vi "Serial_Read_String.vi"(8 "error in (no error)":errorcluster, 11 "VISA Refnum in":refnum<visa-resource-name>) -> (0 "error out":errorcluster, 2 "read buffer":string, 3 "VISA Refnum out":refnum<visa-resource-name>)   [LabVIEW 2020]
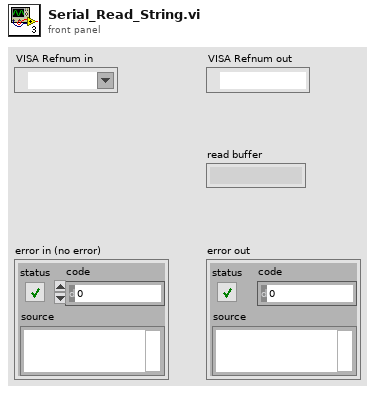
[diagram p1: front panel]
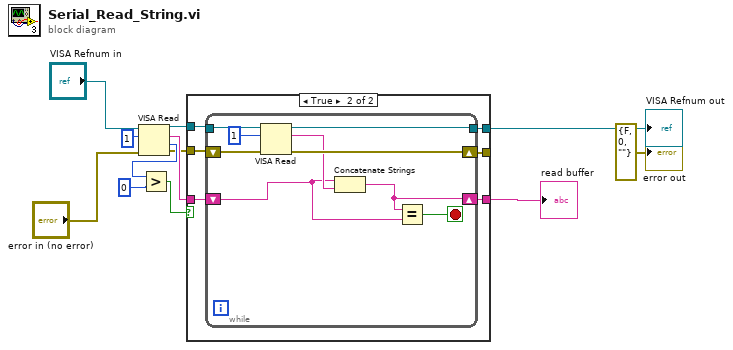
[diagram p0: block diagram]
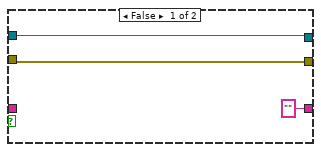
[diagram p2: hidden frame]
diagram:
  n1 = VISA Read(VISA resource name="VISA Refnum in", byte count=u32 1, error in (no error)="error in (no error)") -> (VISA resource name out=w4:refnum<visa-resource-name>, read buffer=w10:string, return count=w11:u32, error out=w5:errorcluster)
  n2 = Greater?(x=w11, y=0) -> (0:w9:bool)
  n3 = case shown="True" w9 {
    tunnel: [w14 w21] -> _
    tunnel: [w15 w20] -> w2
    tunnel: w10 -> [_ w19]
    tunnel: ["" ("read buffer") w18] -> w12
    tunnel: w4 -> [w15 w17]
    tunnel: w5 -> [w14 w16]
    frame False {
    }
    frame True {
      n4 = while {
        tunnel: w17 -> [w30]
        tunnel: [w26] -> w20
        shift-right: [w27] -> w21
        shift-left: w16 -> [w28]
        shift-right: [w23] -> w18
        shift-left: w19 -> [w22]
        stop <- w24 stop-if-true
        n5 = VISA Read(VISA resource name=w30, byte count=u32 1, error in (no error)=w28) -> (VISA resource name out=w26:refnum<visa-resource-name>, read buffer=w25:string, error out=w27:errorcluster)  [unwired: 1 out]
        n6 = Concatenate Strings(w22, w25) -> (w23:string)
        n7 = Equal?(x=w23, y=w22) -> (x = y?=w24:bool)
      }
    }
  }
  "read buffer" <- w12
  "VISA Refnum out" <- w2
  "error out" <- errorcluster {"status"=FALSE, "code"=0, "source"=""} ("error out")
